vi "Get Double.vi"(7 "data type of variable":dbl, 8 "error in":errorcluster, 10 "variable name":string, 11 "GOLPI ref. in":T1={"pipe handle"={"lv_proc.dll file path"=path "", "process instance handle"=[], "debug mode"=FALSE, "debug data"=[]}, "fast read timeout [ms]"=500, "fast read settle time [ms]"=10, "fast read to multiple [ms]"=1, "max elements per input line"=100, "slow read timeout [ms]"=5000, "stdin double format specifier"="%_16e", "max elements per stdout output column"=100, "console mode bitstream"=FALSE, "bitstream first read timeout [ms]"=1000, "bitstream read timeout [ms]"=50, "struct transfer possible"=FALSE, "matlab mode"=FALSE, "var pipe write timeout [ms]"=5000, "variable pipe mode"=FALSE, "variable pipe buffer size [Bytes]"=10000000, "variable pipe block size [Bytes]"=1000000} {"variable pipe block size [Bytes]" format="%.0p"; "variable pipe buffer size [Bytes]" format="%.0p"}) -> (0 "error out":errorcluster, 2 "value":dbl format="%.4g", 3 "GOLPI ref. out":T1={"pipe handle"={"lv_proc.dll file path"=path "", "process instance handle"=[], "debug mode"=FALSE, "debug data"=[]}, "fast read timeout [ms]"=500, "fast read settle time [ms]"=10, "fast read to multiple [ms]"=1, "max elements per input line"=100, "slow read timeout [ms]"=5000, "stdin double format specifier"="%_16e", "max elements per stdout output column"=100, "console mode bitstream"=FALSE, "bitstream first read timeout [ms]"=1000, "bitstream read timeout [ms]"=50, "struct transfer possible"=FALSE, "matlab mode"=FALSE, "var pipe write timeout [ms]"=5000, "variable pipe mode"=FALSE, "variable pipe buffer size [Bytes]"=10000000, "variable pipe block size [Bytes]"=1000000} {"variable pipe block size [Bytes]" format="%.0p"; "variable pipe buffer size [Bytes]" format="%.0p"})   [LabVIEW 2020, in "GOLPI library.lvlib"]
doc: "Part of polymorph Get Variable.vi"
uses:
  GOLPI library.lvlib
  Public/GOLPI reference Type Def.ctl
  LV Process source distribution/Pipe Handle.ctl
  Type Definitions/Custom Error Codes Enum Type Def.vi
  Type Definitions/Bitstream Data Type.ctl
  LV Process source distribution/LV Process library.lvlib
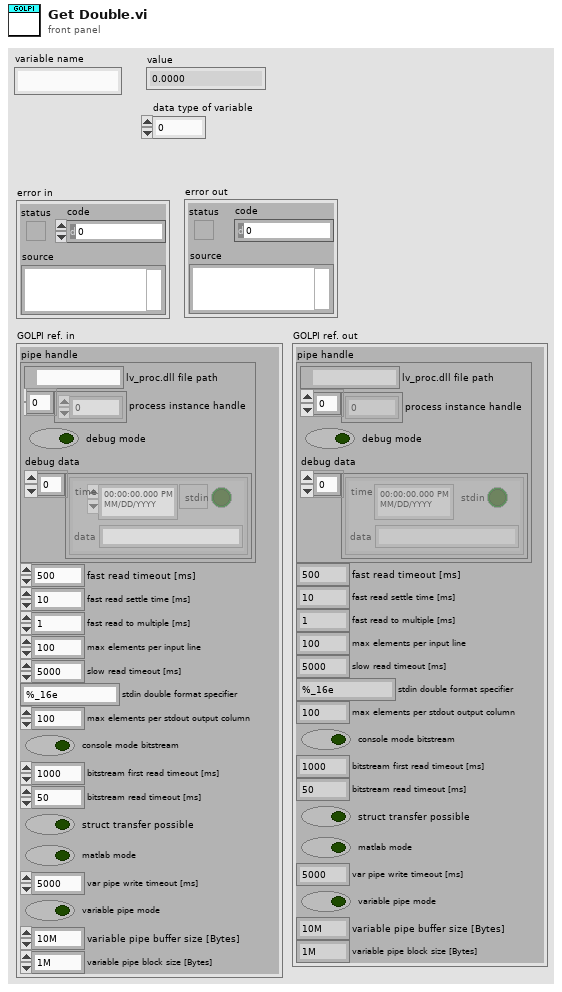
[diagram p1: front panel]
types:
  T1 = typedef "GOLPI library.lvlib/GOLPI reference Type Def.ctl" = cluster{"pipe handle":T2, "fast read timeout [ms]":u32, "fast read settle time [ms]":u32, "fast read to multiple [ms]":u32, "max elements per input line":u32, "slow read timeout [ms]":u32, "stdin double format specifier":string, "max elements per stdout output column":u32, "console mode bitstream":bool, "bitstream first read timeout [ms]":u32, "bitstream read timeout [ms]":u32, "struct transfer possible":bool, "matlab mode":bool, "var pipe write timeout [ms]":u32, "variable pipe mode":bool, "variable pipe buffer size [Bytes]":u32, "variable pipe block size [Bytes]":u32}
  T2 = typedef "LV Process library.lvlib/Pipe Handle.ctl" = cluster{"lv_proc.dll file path":path, "process instance handle":u32[], "debug mode":bool, "debug data":cluster{"time":timestamp, "stdin":bool, "data":string}[]}
  T3 = typedef "GOLPI library.lvlib/Custom Error Codes Enum Type Def.vi" = enum16{"no error", "00 working directory PAR1 missing", "01 octave binary PAR1 missing", "02 octave report error PAR1", "03 empty output last cmd PAR1", "04 missing temporary file PAR1", "05 pwd PAR 1 not exist", "06 oct package not installed", "07 octave default binary missing", "10 var PAR1 not string, vect", "11 var PAR1 not num, scal, ~compl", "12 var PAR1 not num, scal, compl", "13 var PAR1 not num, vect, ~compl", "14 var PAR1 not num, vect, compl", "15 var PAR1 not num, mat, ~compl", "16 var PAR1 not num, mat, ~compl", "30 read timeout", "60 bitstream transport failed", "61 bitstream decode error PAR1", "62 bitstream cannot be set", "70 struct transfer not possible", "80 struct: cluster elem. PAR1 not implem.", "81 struct: structure field PAR1 not implem.", "82 struct: size mismatch of PAR1", "83 struct: type mismatch of PAR1", "98 internal error", "99 not finished", "90 Not supported in Matlab mode", "91 Matlab variable transfer error", "92 Matlab Script Error"}
  T4 = typedef "GOLPI library.lvlib/Bitstream Data Type.ctl" = enum16{"dummy", "int", "uint", "float", "complex", "str", "real numeric"}
  T5 = typedef "GOLPI library.lvlib/Transfer Mode.ctl" = enum16{"Matlab", "stdio", "temp file", "bitstream", "pipe"}
  T6 = typedef "GOLPI library.lvlib/Bitstream Data.ctl" = cluster{"double":dbl[][], "cplx double":cdb[][], "int64":i64[][], "uint64":u64[][], "str":string[], "data type":T4}
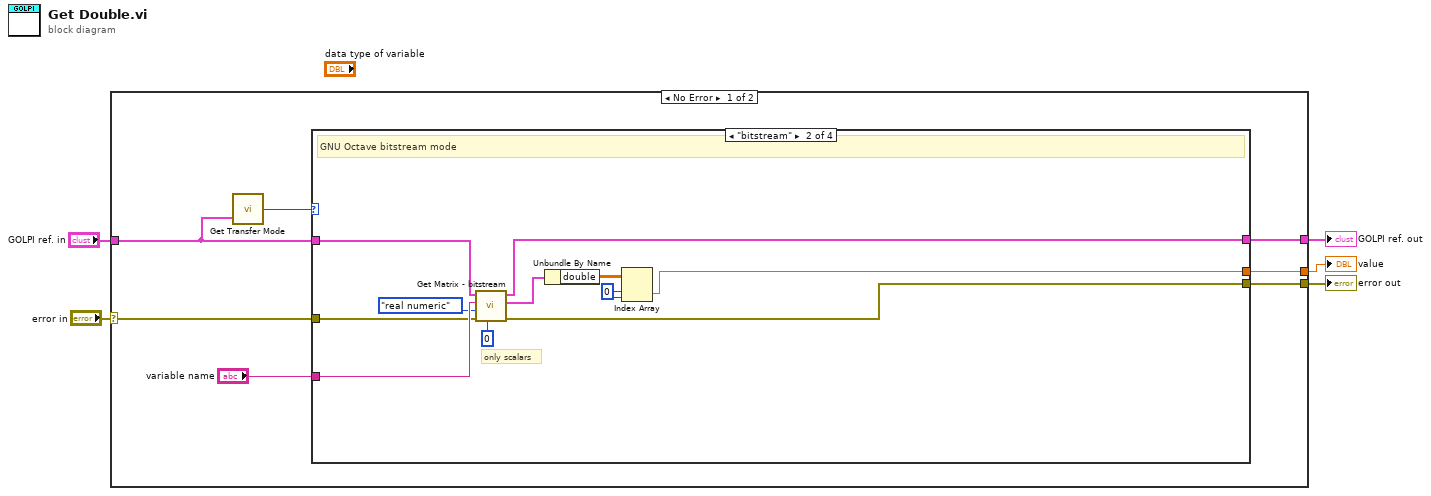
[diagram p0: block diagram]
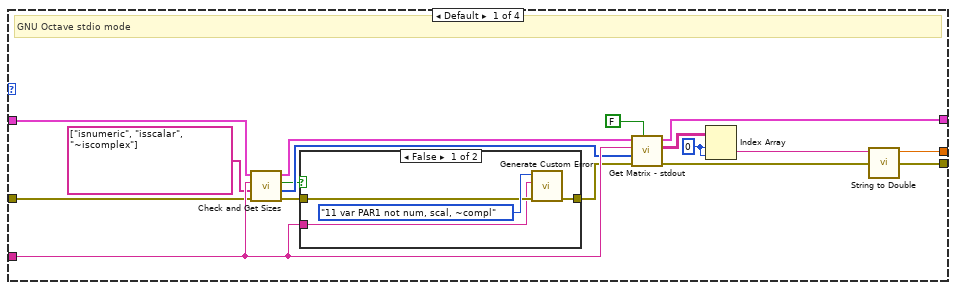
[diagram p2: hidden frame]
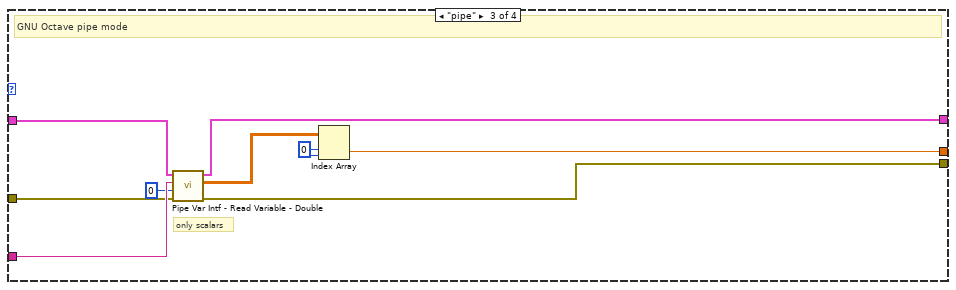
[diagram p4: hidden frame]
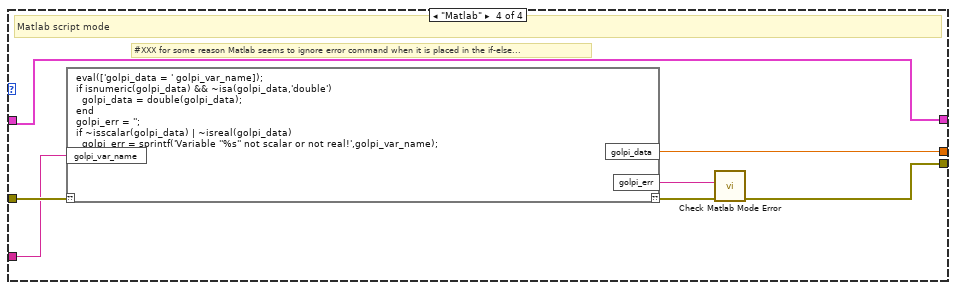
[diagram p5: hidden frame]
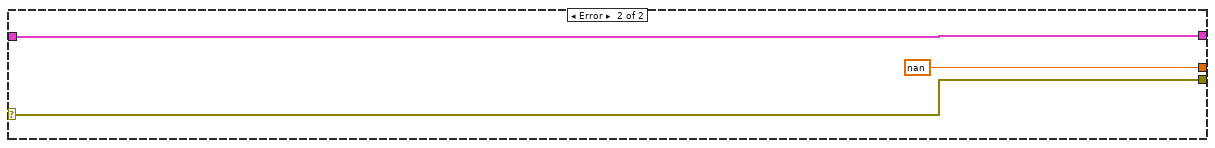
[diagram p6: hidden frame]
diagram:
  n1 = case shown="No Error" "error in" {
    selector: "error in" -> [w10 w63]
    tunnel: [w8 nan ("t")] -> w5
    tunnel: [w9 w63] -> w4
    tunnel: "GOLPI ref. in" -> [w7 w61]
    tunnel: [w11 w61] -> w1
    frame No Error {
      n2 = call "Get Transfer Mode.vi"("GOLPI ref."=w7) -> ("mode"=w6:T5)  [unwired: 1 in]
      n3 = case shown="\"bitstream\"" w6 {
        tunnel: "variable name" -> [w28 w44 w53 w58]
        tunnel: [w27 w43 w52 w59] -> w11
        tunnel: w10 -> [w26 w42 w51 w60]
        tunnel: [w25 w41 w50 w54] -> w9
        tunnel: [w24 w40 w49 w57] -> w8
        tunnel: w7 -> [w23 w39 w48 w59]
        frame Default {
          w17 = 0 ("index (row)")
          # "GNU Octave stdio mode"
          n4 = call "Check and Get Sizes.vi"("error in (no error)"=w26, "test commands"=string[] ["isnumeric", "isscalar", "~iscomplex"], "variable name"=w28, "GOLPI ref. in"=w23) -> ("error out"=w15:errorcluster, "octave sizes"=w21:i32[], "all tests OK?"=w20:bool, "GOLPI ref. out"=w16:T1)  [unwired: 4 in]
          n5 = case shown="False" w20 {
            tunnel: [w30 w33] -> w14
            tunnel: w15 -> [w31 w33]
            tunnel: w28 -> [w29 _]
            frame False {
              n6 = call "Generate Custom Error.vi"("error in"=w31, "PAR1"=w29, "GOLPI error"=Custom_Error_Codes_Enum_Type_Def.vi."11 var PAR1 not num, scal, ~compl" ("Enum")) -> ("error out"=w30:errorcluster)  [unwired: 8 in]
            }
            frame True {
            }
          }
          n7 = call "Get Matrix - stdout.vi"("is string?"=FALSE ("is string"), "error in (no error)"=w14, "octave sizes"=w21, "variable name"=w28, "GOLPI ref. in"=w16) -> ("error out"=w25:errorcluster, "array"=w18:string[][], "GOLPI ref. out"=w27:T1)  [unwired: 4 in]
          n8 = Index Array(array=w18, index (row)=w17, index (col)=w17) -> (element=w13:string)
          n9 = call "String to Double.vi"("string"=w13) -> ("number"=w24:dbl)  [unwired: 10 in]
        }
        frame "bitstream" {
          w34 = 0 ("index (row)")
          # "only scalars"
          # "GNU Octave bitstream mode"
          n10 = call "Get Matrix - bitstream.vi"("max dimensions (0: scalar)"=0, "error in (no error)"=w42, "data type"=Bitstream_Data_Type."real numeric", "variable name"=w44, "GOLPI ref. in"=w39) -> ("error out"=w41:errorcluster, "data"=w36:T6, "GOLPI ref. out"=w43:T1)  [unwired: 4 in]
          n11 = Unbundle By Name(w36) -> ("double"=w35:dbl[][])
          n12 = Index Array(array=w35, index (row)=w34, index (col)=w34) -> (element=w40:dbl)
        }
        frame "pipe" {
          w46 = 0 ("index (row)")
          # "only scalars"
          # "GNU Octave pipe mode"
          n13 = call "Pipe Var Intf - Read Variable - Double.vi"("error in (no error)"=w51, "max dims (0: scalar)"=0 ("max dimensions (0: scalar)"), "variable name"=w53, "GOLPI ref. in"=w48) -> ("error out"=w50:errorcluster, "data out"=w45:dbl[][], "GOLPI ref. out"=w52:T1)  [unwired: 5 in]
          n14 = Index Array(array=w45, index (row)=w46, index (col)=w46) -> (element=w49:dbl)
        }
        frame "Matlab" {
          # "#XXX for some reason Matlab seems to ignore error command when it is placed in the if-else..."
          # "Matlab script mode"
          n15 = script code="eval(['golpi_data = ' golpi_var_name]);\nif isnumeric(golpi_data) && ~isa(golpi_data,'double')\n  golpi_data = double(golpi_data);\nend\ngolpi_err = '';\nif ~isscalar(golpi_data) | ~isreal(golpi_data)\n  golpi_err = sprintf('Variable ''%s'' not scalar or not real!',golpi_var_name);\nend"("??"=w60, "golpi_var_name"=w58) -> ("??"=w56:errorcluster, "golpi_data"=w57:dbl, "golpi_err"=w55:string)
          n16 = call "Check Matlab Mode Error.vi"("error in"=w56, "custom error string (empty)"=w55) -> ("error out"=w54:errorcluster)  [unwired: 9 in]
        }
      }
    }
    frame Error {
    }
  }
  "value" <- w5
  "error out" <- w4
  "GOLPI ref. out" <- w1
